vi "Iteration.vi"(8 "error in (no error)":errorcluster, 11 "Sequence in":refnum<class "Sequence.lvclass">) -> (0 "error out":errorcluster, 1 "Abort":bool, 3 "Sequence out":refnum<class "Sequence.lvclass">)   [LabVIEW 2020, in "VolatusSeq.lvlib" / "Sequence.lvclass"]
uses:
  Sequence.lvclass
  Sequence.lvclass/Sequence.ctl
  State/State.lvclass
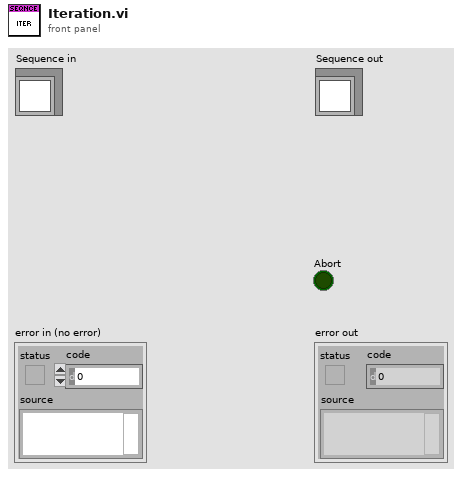
[diagram p1: front panel]
types:
  T1 = typedef "VolatusSeq.lvlib/Iteration Result.ctl" = cluster{"Next State (Current)":string, "Stop":bool, "Abort":bool}
  T2 = typedef "VolatusSeq.lvlib/Sequence Mode.ctl" = enum16{"Unknown", "Loading", "Verifying", "Conflict", "Idle", "Running", "Stopping", "Aborted", "Fault"}
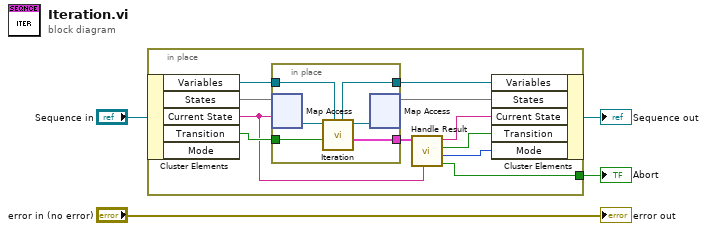
[diagram p0: block diagram]
diagram:
  n1 = in-place {
    in-place-border: [w5] -> w1
    n2 = in-place-cluster #1("Sequence in") -> ("Variables"=w14:refnum<class "Variables.lvclass">, "States"=w15:map{string, refnum<class "State.lvclass">}, "Current State"=w8:string, "Transition"=w11:bool)  [unwired: 1 out]
    n3 = in-place {
      in-place-border: w14 -> [w20]
      in-place-border: [w19] -> w13
      in-place-border: [w17] -> w7
      in-place-border: w11 -> [w16]
      n4 = in-place-map #2(w15, w8) -> (w21:refnum<class "State.lvclass">)  [unwired: 1 in, 1 out]
      n5 = call "Iteration.vi"("Variables in"=w20, "Transition"=w16, "State in"=w21) -> ("Iteration Result"=w17:T1, "State out"=w18:refnum<class "State.lvclass">, "Variables"=w19:refnum<class "Variables.lvclass">)  [unwired: 5 in, 1 out]
      n6 = in-place-map #2(w18) -> (w12:map{string, refnum<class "State.lvclass">})  [unwired: 1 in, 2 out]
    }
    n7 = call "Handle Result.vi"("Prev State"=w8, "Iteration Result"=w7) -> ("Abort"=w5:bool, "Sequence Mode"=w6:T2, "Transition"=w9:bool, "State"=w10:string)  [unwired: 6 in]
    n8 = in-place-cluster #1("Variables"=w13, "States"=w12, "Current State"=w10, "Transition"=w9, "Mode"=w6) -> (→"Sequence out":refnum<class "Sequence.lvclass">)
  }
  "Abort" <- w1
  "error out" <- "error in (no error)"
